vi "Build Dqmh Module Graph.vi"(6 "Draw API Tester Link":bool, 7 "Link Type":T1, 9 "Module Name":string, 10 "Link Name":string[](array[string]), 11 "Graph in":refnum<class "Graph.lvclass">) -> (1 "Specific Edge Shape":T2[](array[typedef]), 2 "Specific Node Shape":T3[](array[typedef]), 3 "Graph out":refnum<class "Graph.lvclass">)   [LabVIEW 2021, in "TAF Proj Document Type.lvlib"]
uses:
  <vilib>/Wovalab/AntiDoc/Document Type/Add-ons/LabVIEW TAF Project/TAF Proj Document Type.lvlib
  <vilib>/Wovalab/AntiDoc/GraphBuilder/Graph/Graph.lvclass
  <vilib>/Wovalab/AntiDoc/GraphBuilder/Renderer/Graphviz/Specific Node Shape Def.ctl
  <vilib>/Wovalab/AntiDoc/GraphBuilder/Shapes/Node/Graphviz/Graphviz Node Shape.lvclass
  <vilib>/Wovalab/AntiDoc/GraphBuilder/Renderer/Graphviz/Specific Edge Shape Def.ctl
  <vilib>/Wovalab/AntiDoc/GraphBuilder/Shapes/Edge/Graphviz/Graphviz Edge Shape.lvclass
  <vilib>/Wovalab/AntiDoc/Document Type/Add-ons/LabVIEW TAF Project/Shared/Dqmh Event Module Link Type.ctl
  <vilib>/Wovalab/AntiDoc/GraphBuilder/Edge/Edge.lvclass
  <vilib>/Wovalab/AntiDoc/GraphBuilder/Node/Node.lvclass
  <vilib>/Wovalab/AntiDoc/GraphBuilder/Shapes/Edge/Graphviz/Shape.ctl
  <vilib>/Wovalab/AntiDoc/GraphBuilder/Renderer/Graphviz/Graphviz.lvclass
  <vilib>/Wovalab/AntiDoc/Utilities/Utilities.lvlib
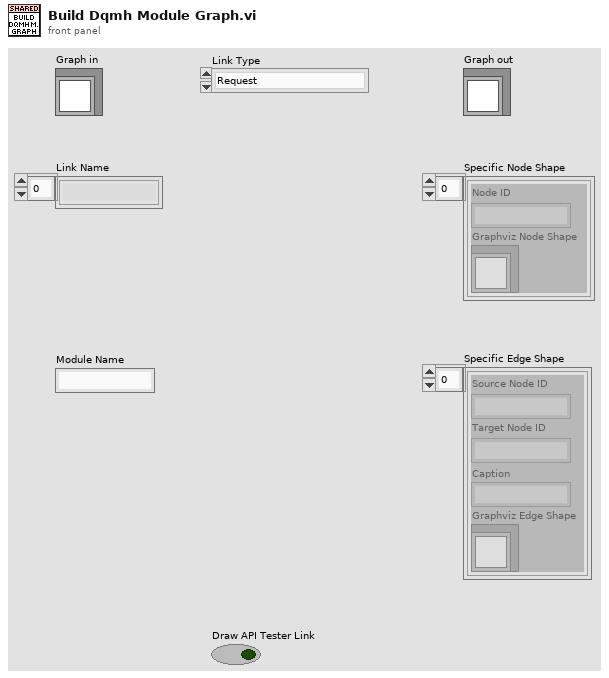
[diagram p1: front panel]
types:
  T1 = typedef "TAF Proj Document Type.lvlib/Dqmh Event Module Link Type.ctl" = enum16{"Request", "Request With Reply", "Broadcast", "Registred Broadcast", "Used Requests", "Used Requests With Reply"}
  T2 = typedef "GraphBuilder.lvlib/Graphviz.lvclass/Specific Edge Shape Def.ctl" = cluster{"Source Node ID":string, "Target Node ID":string, "Caption":string, "Graphviz Edge Shape":refnum<class "Graphviz Edge Shape.lvclass">}
  T3 = typedef "GraphBuilder.lvlib/Graphviz.lvclass/Specific Node Shape Def.ctl" = cluster{"Node ID":string, "Graphviz Node Shape":refnum<class "Graphviz Node Shape.lvclass">}
  T4 = typedef "GraphBuilder.lvlib/Graphviz Edge Shape.lvclass/Shape.ctl" = enum16{"box", "lbox", "rbox", "obox", "olbox", "orbox", "crow", "lcrow", "rcrow", "diamond", "ldiamond", "rdiamond", "odiamond", "oldiamond", "ordiamond", "dot", "odot", "inv", "linv", "rinv", "oinv", "olinv", "orinv", "none", "normal", "lnormal", "rnormal", "onormal", "olnormal", "ornormal", "tee", "ltee", "rtee", "vee", "lvee", "rvee", "curve", "lcurve", "rcurve", "icurve", "licurve", "ricurve"}
  T5 = typedef "GraphBuilder.lvlib/Graphviz Edge Shape.lvclass/Colors.ctl" = enum16{"aliceblue", "antiquewhite", "aqua", "aquamarine", "azure", "beige", "bisque", "black", "blanchedalmond", "blue", "blueviolet", "brown", "burlywood", "cadetblue", "chartreuse", "chocolate", "coral", "cornflowerblue", "cornsilk", "crimson", "cyan", "darkblue", "darkcyan", "darkgoldenrod", "darkgray", "darkgreen", "darkgrey", "darkkhaki", "darkmagenta", "darkolivegreen", "darkorange", "darkorchid", "darkred", "darksalmon", "darkseagreen", "darkslateblue", "darkslategray", "darkslategrey", "darkturquoise", "darkviolet", "deeppink", "deepskyblue", "dimgray", "dimgrey", "dodgerblue", "firebrick", "floralwhite", "forestgreen", "fuchsia", "gainsboro", "ghostwhite", "gold", "goldenrod", "gray", "green", "greenyellow", "grey", "honeydew", "hotpink", "indianred", "indigo", "ivory", "khaki", "lavender", "lavenderblush", "lawngreen", "lemonchiffon", "lightblue", "lightcoral", "lightcyan", "lightgoldenrodyellow", "lightgray", "lightgreen", "lightgrey", "lightpink", "lightsalmon", "lightseagreen", "lightskyblue", "lightslategray", "lightslategrey", "lightsteelblue", "lightyellow", "lime", "limegreen", "linen", "magenta", "maroon", "mediumaquamarine", "mediumblue", "mediumorchid", "mediumpurple", "mediumseagreen", "mediumslateblue", "mediumspringgreen", "mediumturquoise", "mediumvioletred", "midnightblue", "mintcream", "mistyrose", "moccasin", "navajowhite", "navy", "oldlace", "olive", "olivedrab", "orange", "orangered", "orchid", "palegoldenrod", "palegreen", "paleturquoise", "palevioletred", "papayawhip", "peachpuff", "peru", "pink", "plum", "powderblue", "purple", "red", "rosybrown", "royalblue", "saddlebrown", "salmon", "sandybrown", "seagreen", "seashell", "sienna", "silver", "skyblue", "slateblue", "slategray", "slategrey", "snow", "springgreen", "steelblue", "tan", "teal", "thistle", "tomato", "turquoise", "violet", "wheat", "white", "whitesmoke", "yellow", "yellowgreen"}
  T6 = typedef "GraphBuilder.lvlib/Graphviz Edge Shape.lvclass/Style.ctl" = enum8{"filled", "invisible", "diagonals", "rounded", "dashed", "dotted", "solid", "bold"}
  T7 = typedef "GraphBuilder.lvlib/Graphviz Node Shape.lvclass/Shape.ctl" = enum16{"box", "polygon", "ellipse", "oval", "circle", "point", "egg", "triangle", "plaintext", "plain", "diamond", "trapezium", "parallelogram", "house", "pentagon", "hexagon", "septagon", "octagon", "doublecircle", "doubleoctagon", "tripleoctagon", "invtriangle", "invtrapezium", "invhouse", "Mdiamond", "Msquare", "Mcircle", "rect", "rectangle", "square", "star", "none", "underline", "cylinder", "note", "tab", "folder", "box3D", "component", "promoter", "cds", "terminator", "utr", "primersite", "restrictionsite", "fivepoverhang", "threepoverhang", "noverhang", "assembly", "signature", "insulator", "ribosite", "rnastab", "proteasesite", "proteinstab", "rpromoter", "rarrow", "larrow", "lpromoter"}
  T8 = typedef "GraphBuilder.lvlib/Graphviz Node Shape.lvclass/Colors.ctl" = enum16{"aliceblue", "antiquewhite", "aqua", "aquamarine", "azure", "beige", "bisque", "black", "blanchedalmond", "blue", "blueviolet", "brown", "burlywood", "cadetblue", "chartreuse", "chocolate", "coral", "cornflowerblue", "cornsilk", "crimson", "cyan", "darkblue", "darkcyan", "darkgoldenrod", "darkgray", "darkgreen", "darkgrey", "darkkhaki", "darkmagenta", "darkolivegreen", "darkorange", "darkorchid", "darkred", "darksalmon", "darkseagreen", "darkslateblue", "darkslategray", "darkslategrey", "darkturquoise", "darkviolet", "deeppink", "deepskyblue", "dimgray", "dimgrey", "dodgerblue", "firebrick", "floralwhite", "forestgreen", "fuchsia", "gainsboro", "ghostwhite", "gold", "goldenrod", "gray", "green", "greenyellow", "grey", "honeydew", "hotpink", "indianred", "indigo", "ivory", "khaki", "lavender", "lavenderblush", "lawngreen", "lemonchiffon", "lightblue", "lightcoral", "lightcyan", "lightgoldenrodyellow", "lightgray", "lightgreen", "lightgrey", "lightpink", "lightsalmon", "lightseagreen", "lightskyblue", "lightslategray", "lightslategrey", "lightsteelblue", "lightyellow", "lime", "limegreen", "linen", "magenta", "maroon", "mediumaquamarine", "mediumblue", "mediumorchid", "mediumpurple", "mediumseagreen", "mediumslateblue", "mediumspringgreen", "mediumturquoise", "mediumvioletred", "midnightblue", "mintcream", "mistyrose", "moccasin", "navajowhite", "navy", "oldlace", "olive", "olivedrab", "orange", "orangered", "orchid", "palegoldenrod", "palegreen", "paleturquoise", "palevioletred", "papayawhip", "peachpuff", "peru", "pink", "plum", "powderblue", "purple", "red", "rosybrown", "royalblue", "saddlebrown", "salmon", "sandybrown", "seagreen", "seashell", "sienna", "silver", "skyblue", "slateblue", "slategray", "slategrey", "snow", "springgreen", "steelblue", "tan", "teal", "thistle", "tomato", "turquoise", "violet", "wheat", "white", "whitesmoke", "yellow", "yellowgreen"}
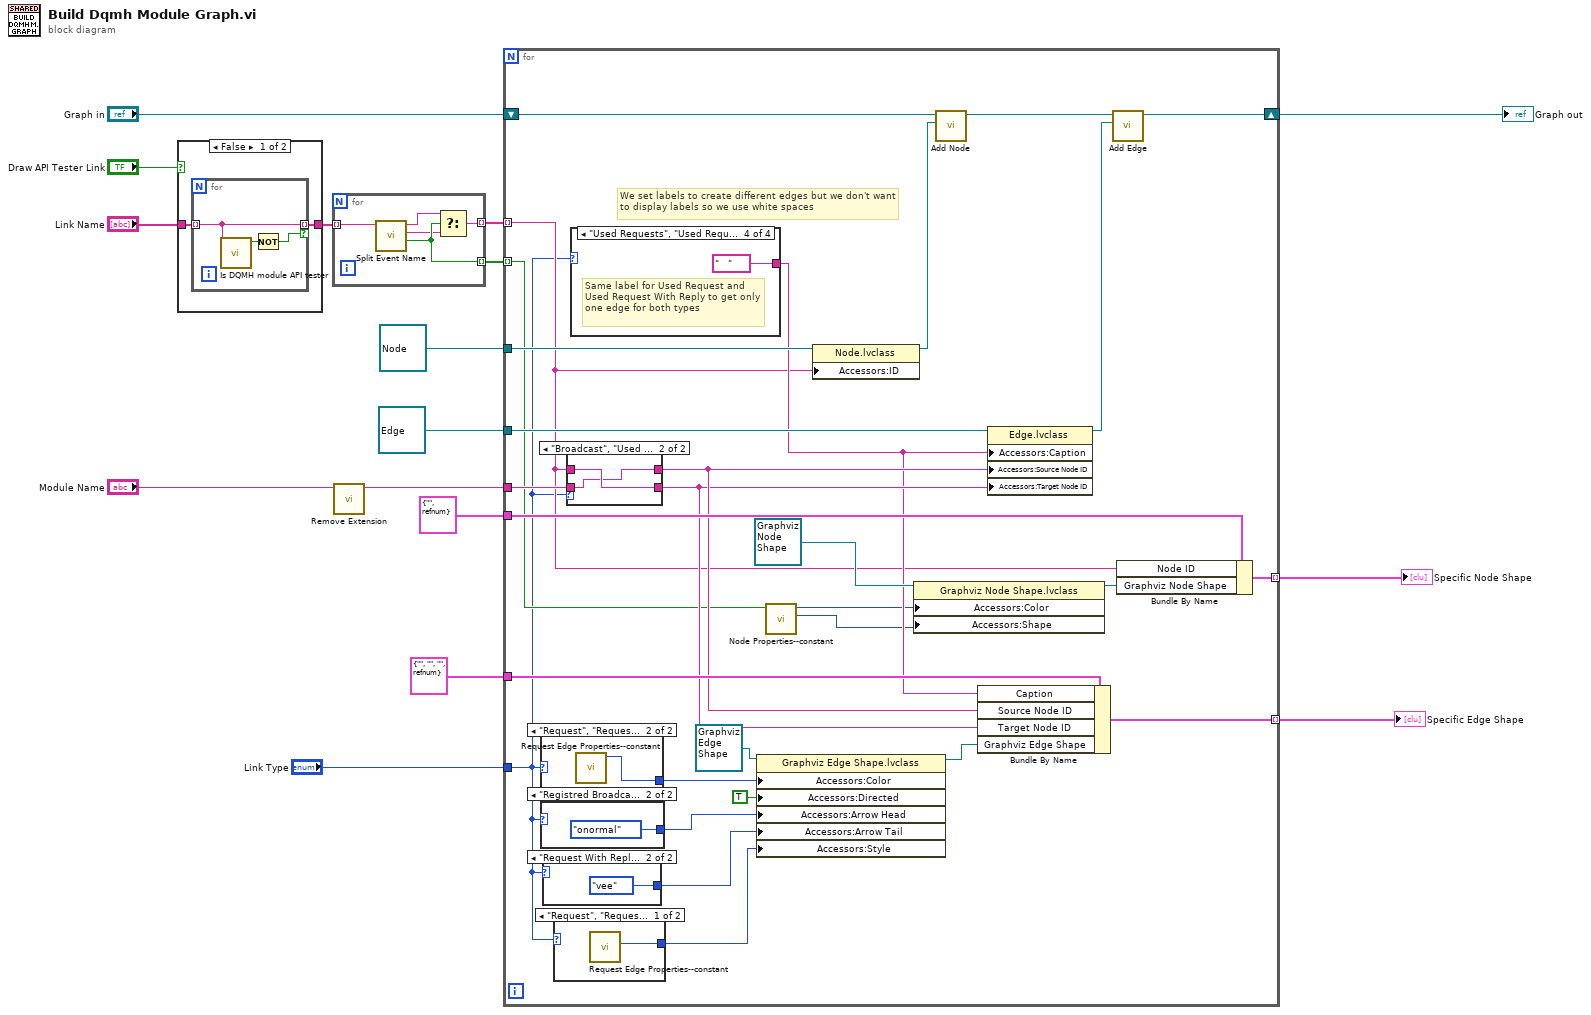
[diagram p0: block diagram]
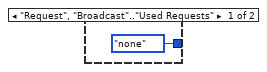
[diagram p3: hidden frame]
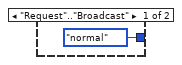
[diagram p4: hidden frame]
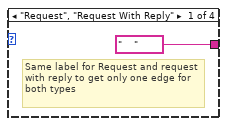
[diagram p5: hidden frame]
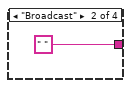
[diagram p6: hidden frame]
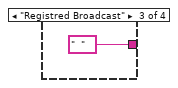
[diagram p7: hidden frame]
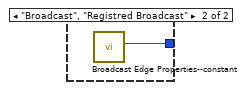
[diagram p8: hidden frame]
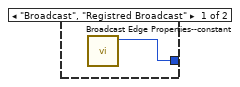
[diagram p10: hidden frame]
diagram:
  n1 = case shown="False" "Draw API Tester Link" {
    tunnel: "Link Name" -> [w18 w22]
    tunnel: [w17 w22] -> w4
    frame False {
      n2 = for {
        tunnel: w18 -> [w21] mode=indexing
        tunnel: [w21] -> w17 mode=indexing if=w19
        n3 = call <vilib>:"Is DQMH module API tester.vi"("File Name"=w21) -> ("Is API Tester?"=w20:bool)  [unwired: 10 in]
        n4 = Not(x=w20) -> (.not. x?=w19:bool)
      }
    }
    frame True {
    }
  }
  n5 = for {
    tunnel: w4 -> [w27] mode=indexing
    tunnel: [w25] -> w6 mode=indexing
    tunnel: [w23] -> w7 mode=indexing
    n6 = call <vilib>:"Split Event Name.vi"("Event Name"=w27) -> ("Lvlib?"=w25:bool, "Vi Name"=w24:string, "Library Name"=w26:string)  [unwired: 8 in]
    n7 = Select(t=w26, s=w25, f=w24) -> (s? t:f=w23:string)
  }
  n8 = call <vilib>:"Remove Extension.vi"("File Name"="Module Name") -> ("File Name Without Extension"=w1:string)  [unwired: 10 in]
  n9 = for {
    shift-right: [w51] -> w9
    shift-left: "Graph in" -> [w56]
    tunnel: refnum<class "Node.lvclass"> refnum ("GraphBuilder.lvlib:Node.lvclass") -> [w55]
    tunnel: refnum<class "Edge.lvclass"> refnum ("GraphBuilder.lvlib:Edge.lvclass") -> [w53]
    tunnel: w1 -> [w37]
    tunnel: T2 {"Source Node ID"="", "Target Node ID"="", "Caption"="", "Graphviz Edge Shape"=refnum} ("Specific Node Shape") -> [w49]
    tunnel: [w46] -> w11 mode=indexing
    tunnel: T3 {"Node ID"="", "Graphviz Node Shape"=refnum} ("Specific Node Shape") -> [w43]
    tunnel: [w41] -> w12 mode=indexing
    tunnel: w7 -> [w29] mode=indexing
    tunnel: w6 -> [w30] mode=indexing
    tunnel: "Link Type" -> [w28]
    # "We set labels to create different edges but we don't want to display labels so we use white spaces"
    n10 = case shown="\"Request\", \"Request With Reply\", \"Used Requests\", \"Used Requests With Reply\"" w28 {
      tunnel: [w71 w72] -> w38
      frame "Broadcast", "Registred Broadcast" {
        n11 = call <vilib>:"Broadcast Edge Properties--constant.vi"() -> ("Edge Color"=w71:T5)  [unwired: 10 in, 1 out]
      }
      frame "Request", "Request With Reply", "Used Requests", "Used Requests With Reply" {
        n12 = call <vilib>:"Request Edge Properties--constant.vi"() -> ("Edge Color"=w72:T5)  [unwired: 10 in, 1 out]
      }
    }
    n13 = case shown="\"Registred Broadcast\"..\"Used Requests With Reply\"" w28 {
      tunnel: [Shape."normal" ("Arrow Head") Shape."onormal" ("Arrow Head")] -> w40
      frame "Request".."Broadcast" {
      }
      frame "Registred Broadcast".."Used Requests With Reply" {
      }
    }
    n14 = case shown="\"Request With Reply\", \"Used Requests With Reply\"" w28 {
      tunnel: [Shape."none" ("Arrow Tail") Shape."vee" ("Arrow Tail")] -> w39
      frame "Request", "Broadcast".."Used Requests" {
      }
      frame "Request With Reply", "Used Requests With Reply" {
      }
    }
    n15 = case shown="\"Request\", \"Request With Reply\", \"Used Requests\", \"Used Requests With Reply\"" w28 {
      tunnel: [w65 w66] -> w34
      frame "Request", "Request With Reply", "Used Requests", "Used Requests With Reply" {
        n16 = call <vilib>:"Request Edge Properties--constant.vi"() -> ("Style"=w65:T6)  [unwired: 10 in, 1 out]
      }
      frame "Broadcast", "Registred Broadcast" {
        n17 = call <vilib>:"Broadcast Edge Properties--constant.vi"() -> ("Style"=w66:T6)  [unwired: 10 in, 1 out]
      }
    }
    n18 = case shown="\"Broadcast\", \"Used Requests\", \"Used Requests With Reply\"" w28 {
      tunnel: [w68 w70] -> w35
      tunnel: w37 -> [w68 w69]
      tunnel: w29 -> [w67 w70]
      tunnel: [w67 w69] -> w36
      frame "Request", "Request With Reply", "Registred Broadcast" {
      }
      frame "Broadcast", "Used Requests", "Used Requests With Reply" {
      }
    }
    n19 = case shown="\"Used Requests\", \"Used Requests With Reply\"" w28 {
      tunnel: ["    " " " "  " "   "] -> w33
      frame "Request", "Request With Reply" {
        # "Same label for Request and request with reply to get only one edge for both types"
      }
      frame "Broadcast" {
      }
      frame "Registred Broadcast" {
      }
      frame "Used Requests", "Used Requests With Reply" {
        # "Same label for Used Request and Used Request With Reply to get only one edge for both types"
      }
    }
    n20 = property class="Graphviz Edge Shape.lvclass"(reference=refnum<class "Graphviz Edge Shape.lvclass"> refnum ("Graphviz Edge Shape"), "Accessors:Color"=w38, "Accessors:Directed"=TRUE ("Directed"), "Accessors:Arrow Head"=w40, "Accessors:Arrow Tail"=w39, "Accessors:Style"=w34) -> (reference out=w47:refnum<class "Graphviz Edge Shape.lvclass">)  [unwired: 1 in, 1 out]
    n21 = call <vilib>:"Node Properties--constant.vi"("Lvlib"=w30) -> ("Shape"=w31:T7, "Color"=w32:T8)  [unwired: 9 in]
    n22 = property class="Node.lvclass"(reference=w55, "Accessors:ID"=w29) -> (reference out=w54:refnum<class "Node.lvclass">)  [unwired: 1 in, 1 out]
    n23 = property class="Graphviz Node Shape.lvclass"(reference=refnum<class "Graphviz Node Shape.lvclass"> refnum ("GraphBuilder.lvlib:Graphviz Node Shape.lvclass"), "Accessors:Color"=w32, "Accessors:Shape"=w31) -> (reference out=w42:refnum<class "Graphviz Node Shape.lvclass">)  [unwired: 1 in, 1 out]
    n24 = call-dynamic "Add Node.vi"("Node"=w54, "Graph in"=w56) -> ("Graph out"=w52:refnum<class "Graph.lvclass">)  [unwired: 8 in, 1 out]
    n25 = Bundle By Name(cluster=w49, "Caption"=w33, "Source Node ID"=w36, "Target Node ID"=w35, "Graphviz Edge Shape"=w47) -> (w46:T2)
    n26 = property class="Edge.lvclass"(reference=w53, "Accessors:Caption"=w33, "Accessors:Source Node ID"=w36, "Accessors:Target Node ID"=w35) -> (reference out=w50:refnum<class "Edge.lvclass">)  [unwired: 1 in, 1 out]
    n27 = call-dynamic "Add Edge.vi"("Edge"=w50, "Graph in"=w52) -> ("Graph out"=w51:refnum<class "Graph.lvclass">)  [unwired: 8 in, 1 out]
    n28 = Bundle By Name(cluster=w43, "Node ID"=w29, "Graphviz Node Shape"=w42) -> (w41:T3)
  }
  "Specific Node Shape" <- w12
  "Specific Edge Shape" <- w11
  "Graph out" <- w9
